vi "LVITX Format Path&Filename TDMS.vi"(2 "filename":string, 3 "path":path) -> (0 "file name without extension":string, 1 "dup file":path)   [LabVIEW 2016, in "LVtoITX.lvclass"]
uses:
  LVtoITX.lvclass
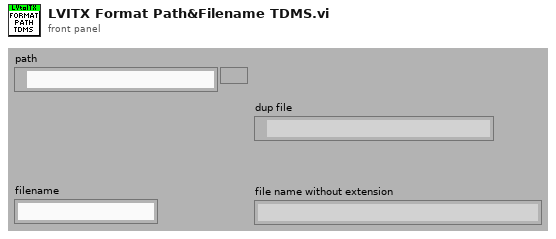
[diagram p1: front panel]
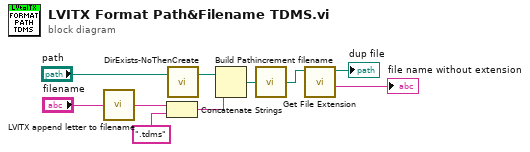
[diagram p0: block diagram]
diagram:
  n1 = call "LVITX append letter to filename.vi"("string in"="filename") -> ("string out"=w1:string)
  n2 = Concatenate Strings(w1, ".tdms" ("string")) -> (w3:string)
  n3 = call <userlib>:"DirExists-NoThenCreate.vi"("path"="path") -> ("created path"=w5:path)  [unwired: 1 in, 1 out]
  n4 = Build Path(base path=w5, name or relative path=w3) -> (appended path=w6:path)
  n5 = call <userlib>:"increment filename.vi"("path"=w6) -> ("modified path"=w4:path)
  n6 = call <vilib>:"Get File Extension.vi"("file"=w4) -> ("filename without extension"=→"file name without extension":string, "dup file"=→"dup file":path)  [unwired: 1 in, 8 out]
